vi "Generate CSV Report.vi"(0 "Serial Number":string, 1 "Date":string, 2 "Time":string, 3 "Retest":string, 4 "Lower Limits":dbl[](array[numeric]), 5 "Measurment values":dbl[](array[numeric]), 6 "Fixture":string, 7 "Upper Limits":dbl[](array[numeric]), 8 "Variant":string, 9 "Status":string[](array[string]), 10 "Project":string, 11 "Overall status":string, 12 "Work Order":string, 13 "Test Names":string[](array[string])) -> (19 "error out":errorcluster)   [LabVIEW 2023, in "CSV Report.lvlib"]
uses:
  CSV Report.lvlib
  <vilib>/Utility/file.llb/Write Delimited Spreadsheet (string).vi
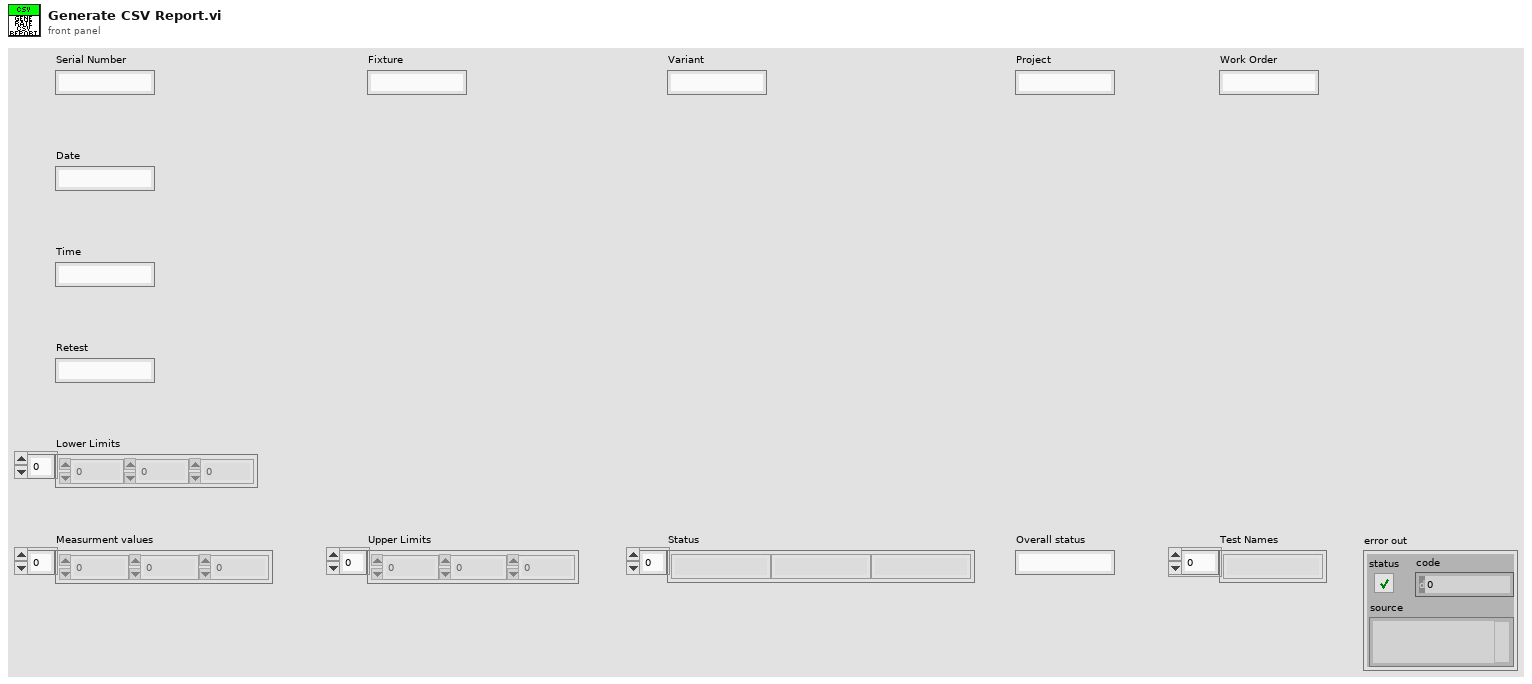
[diagram p1: front panel]
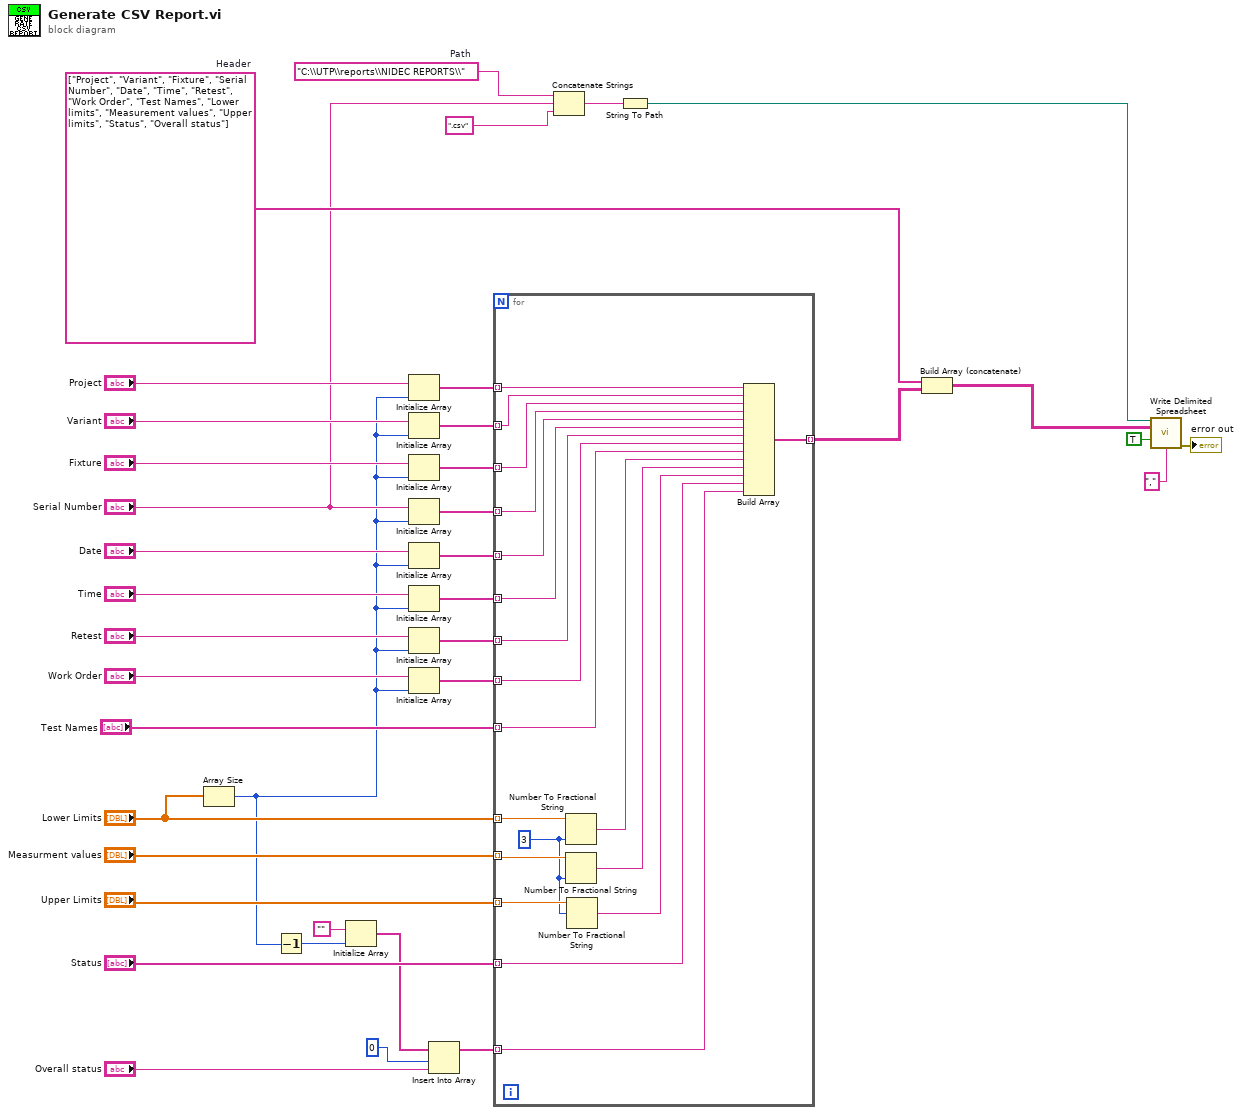
[diagram p0: block diagram]
diagram:
  w22 = "C:\\UTP\\reports\\NIDEC REPORTS\\"  # Path
  w26 = string[] ["Project", "Variant", "Fixture", "Serial Number", "Date", "Time", "Retest", "Work Order", "Test Names", "Lower limits", "Measurement values", "Upper limits", "Status", "Overall status"]  # Header
  n1 = Array Size(array="Lower Limits") -> (size(s)=w3:i32)
  n2 = Decrement(x=w3) -> (x-1=w12:i32)
  n3 = Initialize Array("", w12) -> (w2:string[])
  n4 = Initialize Array("Project", w3) -> (w38:string[])
  n5 = Initialize Array("Variant", w3) -> (w37:string[])
  n6 = Initialize Array("Fixture", w3) -> (w36:string[])
  n7 = Initialize Array("Serial Number", w3) -> (w27:string[])
  n8 = Initialize Array("Date", w3) -> (w35:string[])
  n9 = Initialize Array("Time", w3) -> (w34:string[])
  n10 = Initialize Array("Retest", w3) -> (w23:string[])
  n11 = Initialize Array("Work Order", w3) -> (w9:string[])
  n12 = Insert Into Array(array=w2, index=0, new element="Overall status") -> (w29:string[])
  n13 = for {
    tunnel: w38 -> [w52] mode=indexing
    tunnel: w37 -> [w51] mode=indexing
    tunnel: w36 -> [w50] mode=indexing
    tunnel: w27 -> [w49] mode=indexing
    tunnel: w35 -> [w48] mode=indexing
    tunnel: w34 -> [w47] mode=indexing
    tunnel: "Lower Limits" -> [w57] mode=indexing
    tunnel: "Measurment values" -> [w56] mode=indexing
    tunnel: "Upper Limits" -> [w55] mode=indexing
    tunnel: "Status" -> [w41] mode=indexing
    tunnel: w29 -> [w39] mode=indexing
    tunnel: [w53] -> w25 mode=indexing
    tunnel: w23 -> [w46] mode=indexing
    tunnel: w9 -> [w45] mode=indexing
    tunnel: "Test Names" -> [w40] mode=indexing
    w54 = i16 3 ("precision (6)")
    n14 = Number To Fractional String(number=w57, precision (6)=w54) -> (F-format string=w44:string)  [unwired: 2 in]
    n15 = Number To Fractional String(number=w56, precision (6)=w54) -> (F-format string=w43:string)  [unwired: 2 in]
    n16 = Number To Fractional String(number=w55, width (-)=w54) -> (F-format string=w42:string)  [unwired: 2 in]
    n17 = Build Array(w52, w51, w50, w49, w48, w47, w46, w45, w40, w44, w43, w42, w41, w39) -> (w53:string[])
  }
  n18 = Concatenate Strings(w22, "Serial Number", ".csv" ("string")) -> (w21:string)
  n19 = String To Path(string=w21) -> (path=w20:path)
  n20 = Build Array (concatenate)(w26, w25) -> (w24:string[][])
  n21 = call-poly <vilib>:"Write Delimited Spreadsheet.vi"("file path (dialog if empty)"=w20, "2D data"=w24, "append to file? (new file:F)"=TRUE, "delimiter (\\t)"="," ("delimiter (\\t)")) -> ("error out"=→"error out":errorcluster)  [unwired: 10 in, 1 out]
